vi "Check if Special Steering Frame.vi"(8 "error in (no error)":errorcluster, 11 "special steering frame in":refnum<class "NI_Robotics_Special Steering Frame.lvclass">) -> (0 "error out":errorcluster, 2 "special?":bool, 3 "special steering frame out":refnum<class "NI_Robotics_Special Steering Frame.lvclass">)   [LabVIEW 2017, in "NI_Robotics_Special Steering Frame.lvclass"]
uses:
  <vilib>/robotics/Steering/Special Steering Frame/NI_Robotics_Special Steering Frame.lvclass
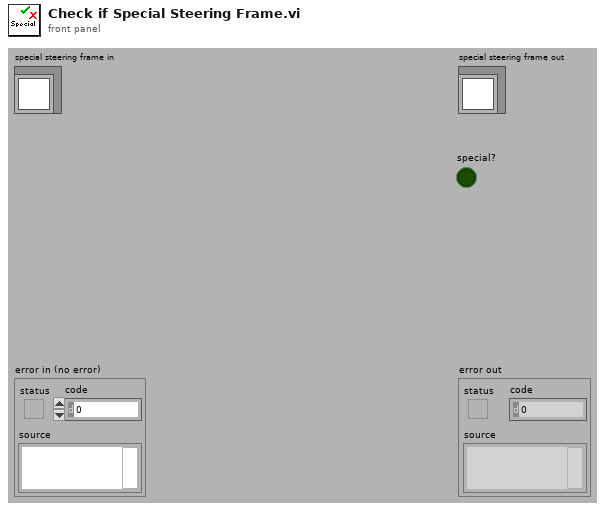
[diagram p1: front panel]
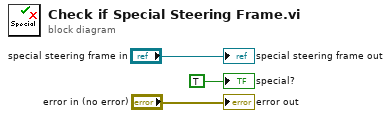
[diagram p0: block diagram]
diagram:
  "error out" <- "error in (no error)"
  "special steering frame out" <- "special steering frame in"
  "special?" <- TRUE ("Special")
